vi "dfd_Modify Hogenauer Bj.vi"(6 "Threshold (< 1)":dbl, 7 "modify?":bool, 9 "Fj":dbl[](array[numeric]), 11 "Hogenauer Bj":i32[](array[numeric])) -> (1 "sum":dbl, 3 "output Bj":i32[](array[numeric]))   [LabVIEW 2017, in "NI_DigFilter_FXP.lvlib"]
uses:
  <vilib>/addons/Digital Filter Design/NI_DigFilter_FXP.lvlib
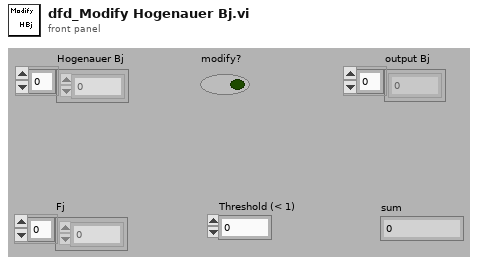
[diagram p1: front panel]
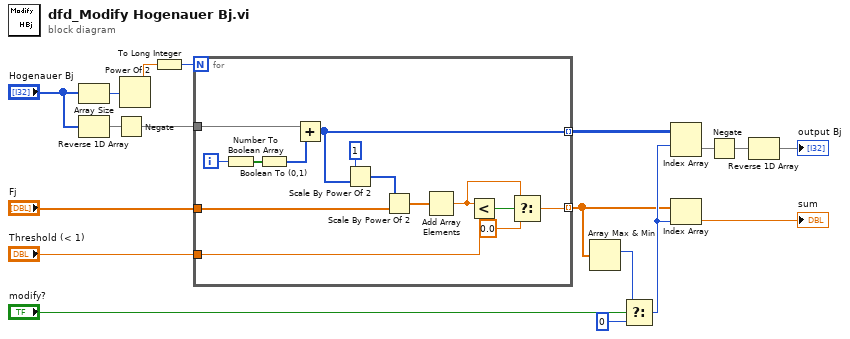
[diagram p0: block diagram]
diagram:
  n1 = Array Size(array="Hogenauer Bj") -> (size(s)=w5:i32)
  n2 = Reverse 1D Array(array="Hogenauer Bj") -> (reversed array=w18:i32[])
  n3 = Negate(x=w18) -> (-x=w15:i32[])
  n4 = Power Of 2(x=w5) -> (2^x=w16:dbl)
  n5 = To Long Integer(number=w16) -> (32bit integer=w3:i32)
  n6 = for {
    N: w3 -> [_]
    tunnel: w15 -> [w30]
    tunnel: "Fj" -> [w26]
    tunnel: [w28] -> w12 mode=indexing
    tunnel: "Threshold (< 1)" -> [w23]
    tunnel: [w19] -> w4 mode=indexing
    i -> [w32]
    n7 = Number To Boolean Array(number=w32) -> (Boolean array=w31:bool[])
    n8 = Boolean To (0,1)(Boolean=w31) -> (0, 1=w29:i16[])
    n9 = Add(x=w30, y=w29) -> (x+y=w28:i32[])
    n10 = Scale By Power Of 2(n=1, x=w28) -> (x*2^n=w25:i32[])
    n11 = Scale By Power Of 2(n=w25, x=w26) -> (x*2^n=w24:dbl[])
    n12 = Add Array Elements(numeric array=w24) -> (sum=w21:dbl)
    n13 = Less?(x=w21, y=w23) -> (x < y?=w22:bool)
    n14 = Select(t=w21, s=w22, f=0.0) -> (s? t:f=w19:dbl)
  }
  n15 = Array Max & Min(array=w4) -> (max index (indices)=w1:i32)  [unwired: 3 out]
  n16 = Select(t=w1, s="modify?", f=0) -> (s? t:f=w9:i32)
  n17 = Index Array(array=w12, index (row)=w9) -> (element=w8:i32[])  [unwired: 1 in]
  n18 = Index Array(array=w4, index=w9) -> (element=→"sum":dbl)
  n19 = Negate(x=w8) -> (-x=w7:i32[])
  n20 = Reverse 1D Array(array=w7) -> (reversed array=→"output Bj":i32[])
